vi "Adjust Center Wavelength.vi"(9 "Polynomial Coefficients in":dbl[](array[numeric]), 10 "Spectrometer Wavelength":dbl, 11 "Numeric":dbl) -> (3 "Polynomial Coefficients out":dbl[](array[numeric]))   [LabVIEW 2020, in "Spectrometer Calibration.lvlib"]
uses:
  Spectrometer Calibration.lvlib
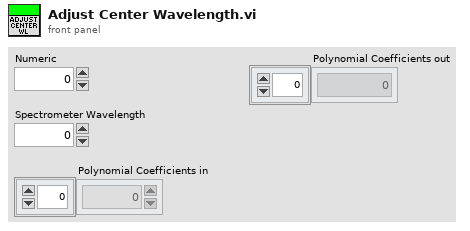
[diagram p1: front panel]
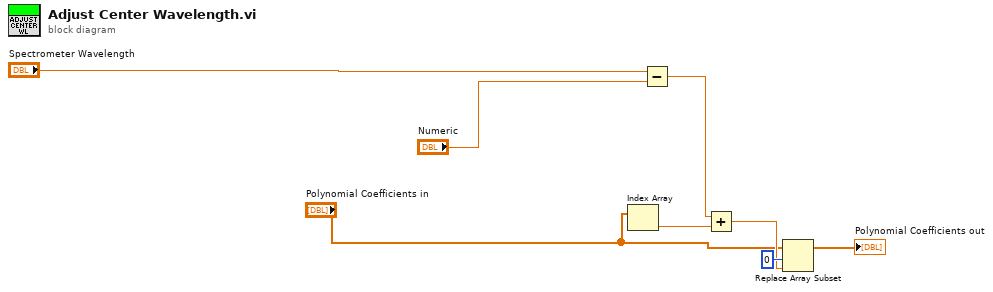
[diagram p0: block diagram]
diagram:
  n1 = Index Array(array="Polynomial Coefficients in") -> (element=w7:dbl)  [unwired: 1 in]
  n2 = Subtract(x="Spectrometer Wavelength", y="Numeric") -> (x-y=w8:dbl)
  n3 = Add(x=w8, y=w7) -> (x+y=w4:dbl)
  n4 = Replace Array Subset(array="Polynomial Coefficients in", new element=w4, index=0) -> (→"Polynomial Coefficients out":dbl[])
